vi "DAQ꾸르잼.vi"() -> ()   [LabVIEW 2018]
uses:
  <vilib>/DAQmx/read.llb/DAQmx Read (Analog Wfm 1Chan NSamp).vi
  <vilib>/DAQmx/create/channels.llb/DAQmx Create Channel (AI-Voltage-Basic).vi
  <vilib>/DAQmx/configure/timing.llb/DAQmx Timing (Sample Clock).vi
  <vilib>/DAQmx/miscellaneous.llb/DAQmx Fill In Error Info.vi
  <vilib>/express/express analysis/Spectral/Block/exnSpectralBlock spectral measurements power poly.vi
  <vilib>/express/express analysis/Spectral/Block/exnSpectralBlock spectral measurements power WFM.vi
  <vilib>/express/express analysis/Spectral/XNode/ExpressSpectralMeasurementsBlockNode.xnode
panel:
  out "웨이브폼 그래프":cluster{"f0":dbl, "df":dbl, "magnitude":dbl[]}(graph)
  out "주파수":dbl
  in  "정지 버튼":bool
  in  "number of samples per channel":i32=-1 caption="채널당 샘플 개수"
  in  "samples per channel":i32=1000 caption="채널당 샘플"
  in  "sample mode":i32(ring)=10178 caption="샘플 모드" items=["유한 샘플"=10178, "연속 샘플"=10123, "하드웨어 타이밍에 의한 단일 포인트"=12522]
  in  "rate":dbl=1000.0 caption="속도" format="%0.2f"
  out "data":waveform(dbl)(graph)
  in  "timeout":dbl=10.0 caption="타임아웃" format="%0.2f"
  in  "input terminal configuration":i32(ring)=-1 caption="입력 터미널 설정" items=["기본"=-1, "RSE"=10083, "NRSE"=10078, "차동"=10106, "유사 차동"=12529]
  in  "minimum value":dbl=-5.0 caption="최소값" format="%0.2f"
  in  "maximum value":dbl=5.0 caption="최대값" format="%0.2f"
  in  "physical channels":tag caption="물리적 채널"
  in  "name to assign":string caption="할당된 이름"
  in  "error in":errorcluster caption="에러 입력"
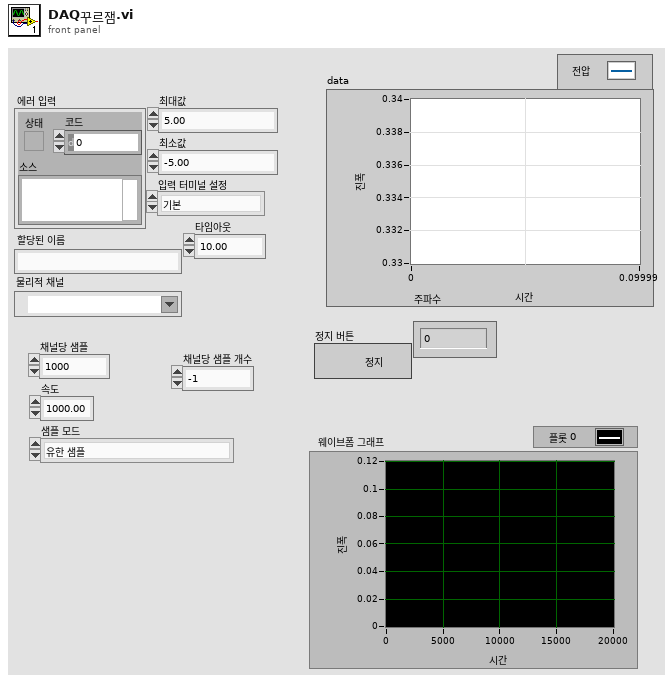
[diagram p1: front panel]
types:
  T1 = cluster{"averaging mode":u16, "weighting mode":u16, "number of averages":u32}
  T2 = cluster{"dB On (F)":bool, "unwrap phase (F)":bool, "convert to degree (F)":bool}
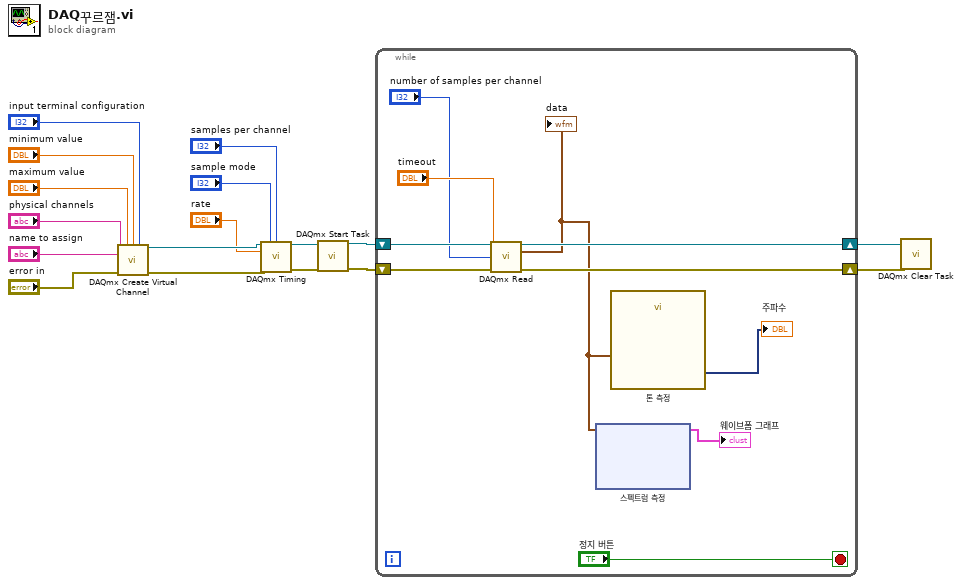
[diagram p0: block diagram]
diagram:
  n1 = call-poly <vilib>:"DAQmx Create Virtual Channel.vi"("maximum value"="maximum value", "minimum value"="minimum value", "input terminal configuration"="input terminal configuration", "physical channels"="physical channels", "name to assign"="name to assign", "error in"="error in") -> ("task out"=w7:refnum<k21>, "error out"=w5:errorcluster)  [unwired: 8 in]
  n2 = call-poly <vilib>:"DAQmx Timing.vi"("task/channels in"=w7, "sample mode"="sample mode", "samples per channel"="samples per channel", "rate"="rate", "error in"=w5) -> ("task out"=w6:refnum<k21>, "error out"=w4:errorcluster)  [unwired: 9 in]
  n3 = call <vilib>:"DAQmx Start Task.vi"("task/channels in"=w6, "error in"=w4) -> ("task out"=w11:refnum<k21>, "error out"=w10:errorcluster)  [unwired: 12 in]
  n4 = while {
    shift-right: [w24] -> w9
    shift-left: w11 -> [w27]
    shift-right: [w23] -> w8
    shift-left: w10 -> [w26]
    stop <- "정지 버튼" stop-if-true
    n5 = call-poly <vilib>:"DAQmx Read.vi"("task/channels in"=w27, "number of samples per channel"="number of samples per channel", "timeout"="timeout", "error in"=w26) -> ("task out"=w24:refnum<k21>, "data"=w20:waveform(dbl), "error out"=w23:errorcluster)  [unwired: 9 in]
    "data" <- w20
    n6 = xnode "스펙트럼 측정"("신호"=w20) -> ("파워 스펙트럼"=→"웨이브폼 그래프":cluster{"f0":dbl, "df":dbl, "magnitude":dbl[]})  [unwired: 1 in, 1 out]
    n7 = call "톤 측정"("Signals"=w20) -> ("Frequency"=→"주파수":dynamicdata)  [unwired: 9 in, 1 out]
  }
  n8 = call <vilib>:"DAQmx Clear Task.vi"("task in"=w9, "error in"=w8) -> ()  [unwired: 13 in, 1 out]
